vi "Cmd-Rec Get Data.vi"(4 "error in (no error)":errorcluster, 7 "command-recordset reference":T4) -> (0 "error out":errorcluster, 1 "object is locked?":bool, 2 "data":T1, 3 "command-recordset reference out":T4)   [LabVIEW 2013, in "NI_Database_API_64.lvlib"]
doc: "Returns a cluster containing the separate Command and Recordset object references of a <B>Command-Recordset</B> object.\n\nIf the object is currently locked for modification, <B>object is locked?</B> will return TRUE.\n\n[GOOP 1.0/1.0]"
uses:
  NI_Database_API_64.lvlib
  Cmd-Rec Data Members.ctl
  Recordset.llb/Rec ObjectReference.ctl
  Command.llb/Cmd ObjectReference.ctl
  Cmd-Rec Object Reference.ctl
  <vilib>/Utility/_goopsup.llb/GOOP Object Repository Method.ctl
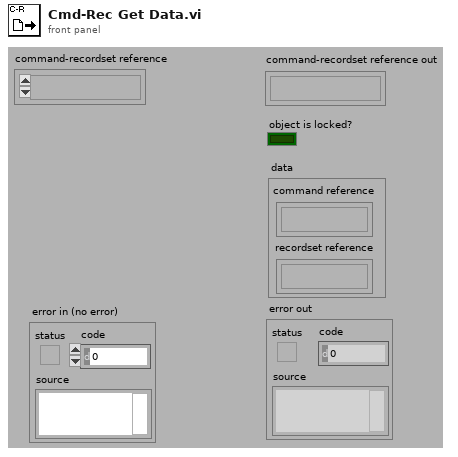
[diagram p1: front panel]
types:
  T1 = typedef "NI_Database_API_64.lvlib/Cmd-Rec Data Members.ctl" = cluster{"recordset reference":T2, "command reference":T3}
  T2 = typedef "NI_Database_API_64.lvlib/Rec ObjectReference.ctl" = refnum<k1>
  T3 = typedef "NI_Database_API_64.lvlib/Cmd ObjectReference.ctl" = refnum<k1>
  T4 = typedef "NI_Database_API_64.lvlib/Cmd-Rec Object Reference.ctl" = refnum<k1>
  T5 = typedef "GOOP Object Repository Method.ctl" = enum16{"Create", "GetCopy", "GetModify", "Set", "Destroy", "Create Static", "Get All Refs", "Reset", "Get Statistics"}
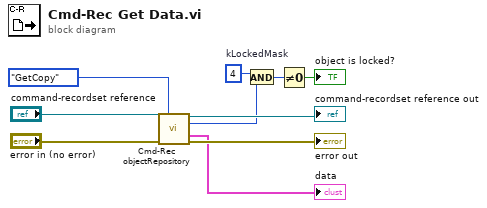
[diagram p0: block diagram]
diagram:
  w3 = 4  # kLockedMask
  n1 = call "Cmd-Rec objectRepository.vi"("command-recordset reference"="command-recordset reference", "method"=GOOP_Object_Repository_Method."GetCopy", "error in (no error)"="error in (no error)") -> ("command-recordset reference out"=→"command-recordset reference out":T4, "flags out"=w2:i32, "classDataOut"=→"data":T1, "error out"=→"error out":errorcluster)  [unwired: 6 in, 3 out]
  n2 = And(x=w3, y=w2) -> (x .and. y?=w4:i32)
  n3 = Not Equal To 0?(x=w4) -> (x != 0?=→"object is locked?":bool)
